vi "Display Welcome User.vi"(8 "error in (no error)":errorcluster, 10 "Sign(Ref)":refnum<vi>, 11 "Admin_Actor in":refnum<class "Admin_Actor.lvclass">) -> (0 "error out":errorcluster, 3 "Admin_Actor out":refnum<class "Admin_Actor.lvclass">)   [LabVIEW 2015, in "Admin_Actor.lvlib" / "Admin_Actor.lvclass"]
uses:
  Admin_Actor.lvclass
  Admin_Actor.lvclass/Admin_Actor.ctl
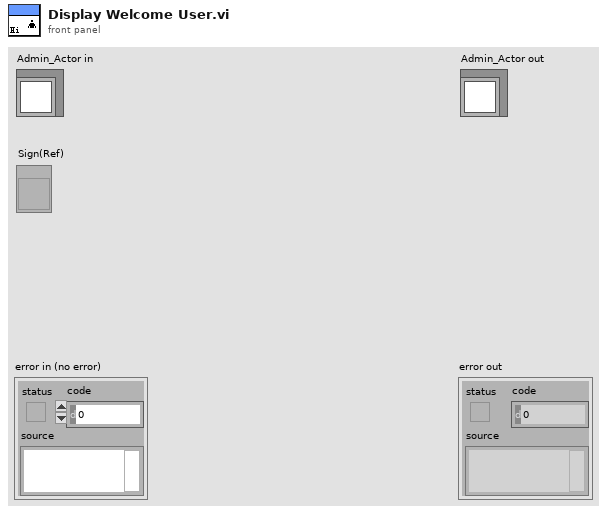
[diagram p1: front panel]
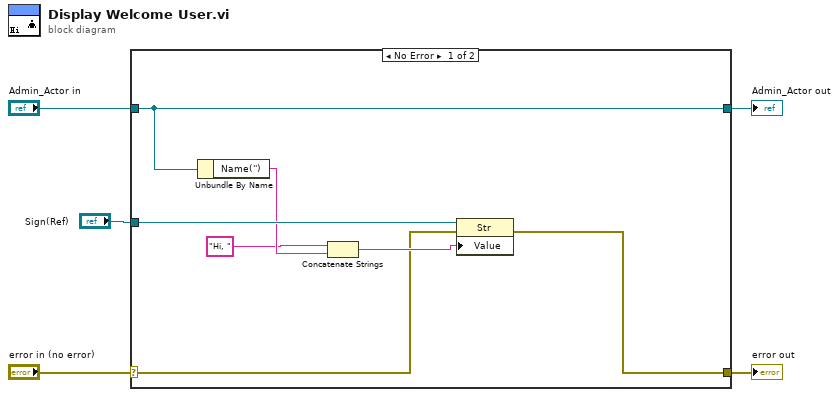
[diagram p0: block diagram]
diagram:
  n1 = case shown="No Error" "error in (no error)" {
    selector: "error in (no error)" -> [w7 w14]
    tunnel: [w6 w14] -> w4
    tunnel: [w12 w13] -> w2
    tunnel: "Admin_Actor in" -> [w12 w13]
    tunnel: "Sign(Ref)" -> [w11 _]
    frame No Error {
      n2 = Unbundle By Name(w12) -> ("Name('')"=w10:string)
      n3 = Concatenate Strings("Hi, " ("string"), w10) -> (w8:string)
      n4 = property class="Str"(reference=w11, error in=w7, "Value"=w8) -> (error out=w6:errorcluster)  [unwired: 1 out]
    }
    frame Error {
    }
  }
  "error out" <- w4
  "Admin_Actor out" <- w2
